vi "KGN Set Pump Mode.vi"(7 "PumpMode-Cluster":T3(array[cluster]) {"concentratio mode" items=["water", "reagent"]; "Reagent" items=["HCl", "HF", "NH3", "HG", "PPM", "ORGANIC"]}, 8 "Fehler (Eingang, kein Fehler)":errorcluster, 9 "Info Cluster":T4, 10 "VISA-Referenz (Eingang)":refnum<visa-resource-name>, 11 "device (Eingang)":u32) -> (0 "Fehler (Ausgang)":errorcluster, 1 "Info Cluster out":T4, 2 "VISA-Referenz (Ausgang)":refnum<visa-resource-name>, 3 "dup device (Ausgang)":u32, 4 "Kommandos gesendet":string[](array[string]))   [LabVIEW 2020, in "Linearisierung v2.lvlib" / "Gasteiler.lvlib" / "HovaCAL_Interface.lvlib" / "KGN.lvlib" / "KGN GUI Set.lvlib"]
uses:
  KGN GUI Set.lvlib
  Controls/Info Cluster.ctl
  Controls/Pump Concentration Mode.ctl
  Controls/Reagent.ctl
  set/set.lvlib
  Controls/Controls.lvlib
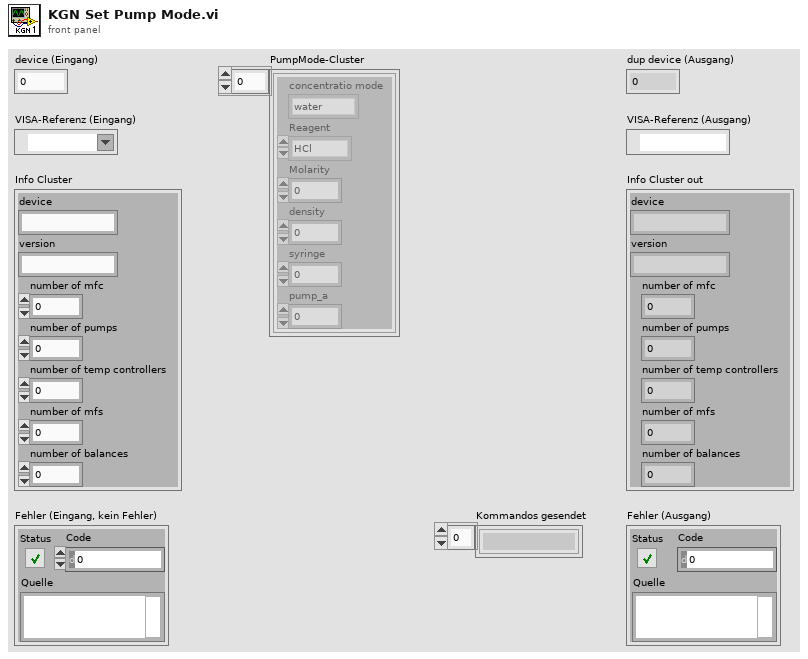
[diagram p1: front panel]
types:
  T1 = typedef "Linearisierung v2.lvlib/Gasteiler.lvlib/HovaCAL_Interface.lvlib/Controls.lvlib/Pump Concentration Mode.ctl" = i32
  T2 = typedef "Linearisierung v2.lvlib/Gasteiler.lvlib/HovaCAL_Interface.lvlib/Controls.lvlib/Reagent.ctl" = i32
  T3 = cluster{"concentratio mode":T1, "Reagent":T2, "Molarity":dbl, "density":dbl, "syringe":dbl, "pump_a":dbl}[]
  T4 = typedef "Linearisierung v2.lvlib/Gasteiler.lvlib/HovaCAL_Interface.lvlib/Controls.lvlib/Info Cluster.ctl" = cluster{"device":string, "version":string, "number of mfc":i32, "number of pumps":i32, "number of temp controllers":i32, "number of mfs":i32, "number of balances":i32}
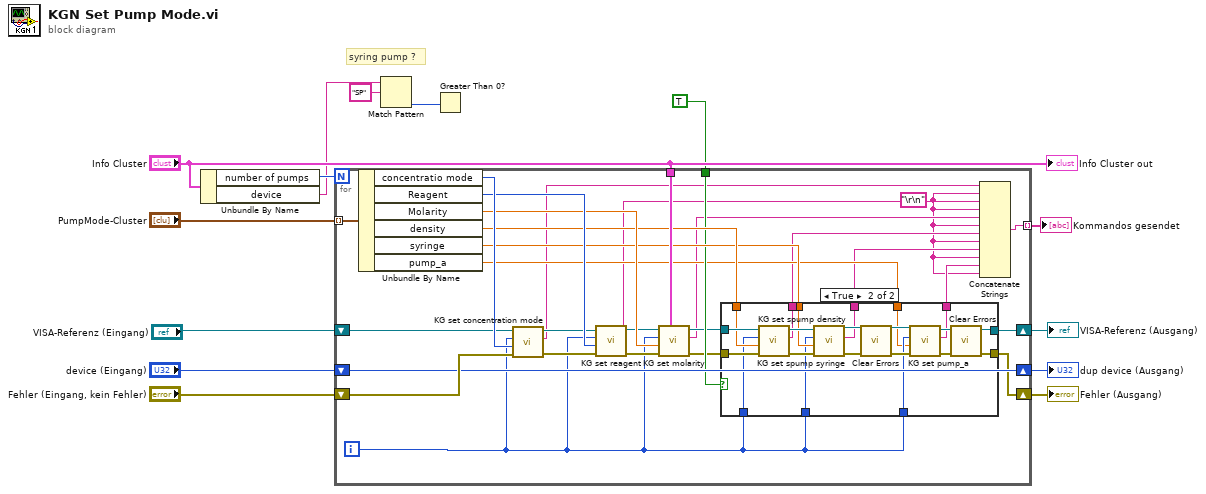
[diagram p0: block diagram]
diagram:
  # "syring pump ?"
  n1 = Unbundle By Name("Info Cluster") -> ("number of pumps"=w9:i32, "device"=w3:string)
  n2 = for {
    N: w9 -> [_]
    tunnel: "PumpMode-Cluster" -> [w42] mode=indexing
    shift-right: [w39] -> w11
    shift-left: "device (Eingang)" -> [w39]
    shift-right: [w38] -> w10
    shift-left: "Fehler (Eingang, kein Fehler)" -> [w43]
    shift-right: [w35] -> w7
    shift-left: "VISA-Referenz (Eingang)" -> [w36]
    tunnel: "Info Cluster" -> [w34]
    tunnel: TRUE -> [w31]
    tunnel: [w16] -> w1 mode=indexing
    i -> [w24]
    w15 = "\r\n"
    n3 = Unbundle By Name(w42) -> ("concentratio mode"=w41:T1, "Reagent"=w40:T2, "Molarity"=w37:dbl, "density"=w33:dbl, "syringe"=w32:dbl, "pump_a"=w23:dbl)
    n4 = call "KG set concentration mode.vi"("Fehler (Eingang, kein Fehler)"=w43, "mode"=w41, "pump"=w24, "VISA-Ressourcenname"=w36) -> ("Fehler (Ausgang)"=w27:errorcluster, "Kommando gesendet"=w22:string, "VISA-Ressourcenname (Ausgang)"=w30:refnum<visa-resource-name>)  [unwired: 5 in]
    n5 = call "KG set reagent.vi"("Fehler (Eingang, kein Fehler)"=w27, "reagent"=w40, "pump"=w24, "VISA-Ressourcenname"=w30) -> ("Fehler (Ausgang)"=w28:errorcluster, "Kommando gesendet"=w21:string, "VISA-Ressourcenname (Ausgang)"=w29:refnum<visa-resource-name>)  [unwired: 5 in]
    n6 = call "KG set molarity.vi"("Info Cluster"=w34, "Fehler (Eingang, kein Fehler)"=w28, "molarity"=w37, "pump"=w24, "VISA-Ressourcenname"=w29) -> ("Fehler (Ausgang)"=w25:errorcluster, "Kommando gesendet"=w20:string, "VISA-Ressourcenname (Ausgang)"=w26:refnum<visa-resource-name>)  [unwired: 4 in]
    n7 = case shown="True" w31 {
      tunnel: [w45 w53] -> w35
      tunnel: w26 -> [w45 w63]
      tunnel: w25 -> [w44 w62]
      tunnel: [w44 w55] -> w38
      tunnel: w33 -> [_ w60]
      tunnel: w32 -> [_ w59]
      tunnel: w24 -> [_ w58]
      tunnel: w24 -> [_ w57]
      tunnel: w24 -> [_ w50]
      tunnel: w23 -> [_ w49]
      tunnel: [_ w48] -> w19
      tunnel: [_ w47] -> w18
      tunnel: [_ w46] -> w17
      frame False {
      }
      frame True {
        n8 = call "KG set spump density.vi"("Fehler (Eingang, kein Fehler)"=w62, "density"=w60, "pump"=w57, "VISA-Ressourcenname"=w63) -> ("Fehler (Ausgang)"=w61:errorcluster, "Kommando gesendet"=w48:string, "VISA-Ressourcenname (Ausgang)"=w64:refnum<visa-resource-name>)  [unwired: 5 in]
        n9 = call "KG set spump syringe.vi"("Fehler (Eingang, kein Fehler)"=w61, "density"=w59, "pump"=w58, "VISA-Ressourcenname"=w64) -> ("Fehler (Ausgang)"=w56:errorcluster, "Kommando gesendet"=w47:string, "VISA-Ressourcenname (Ausgang)"=w54:refnum<visa-resource-name>)  [unwired: 5 in]
        n10 = call <vilib>:"Clear Errors.vi"("error in (no error)"=w56) -> ("error out"=w51:errorcluster)  [unwired: 5 in, 1 out]
        n11 = call "KG set pump_a.vi"("Fehler (Eingang, kein Fehler)"=w51, "A"=w49, "pump"=w50, "VISA-Ressourcenname"=w54) -> ("Fehler (Ausgang)"=w52:errorcluster, "Kommando gesendet"=w46:string, "VISA-Ressourcenname (Ausgang)"=w53:refnum<visa-resource-name>)  [unwired: 5 in]
        n12 = call <vilib>:"Clear Errors.vi"("error in (no error)"=w52) -> ("error out"=w55:errorcluster)  [unwired: 5 in, 1 out]
      }
    }
    n13 = Concatenate Strings(w22, w15, w21, w15, w20, w15, w19, w15, w18, w15, w17, w15) -> (w16:string)
  }
  "dup device (Ausgang)" <- w11
  "Fehler (Ausgang)" <- w10
  "VISA-Referenz (Ausgang)" <- w7
  "Kommandos gesendet" <- w1
  n14 = Match Pattern(string=w3, regular expression="SP" ("Regulärer Ausdruck")) -> (offset past match=w4:i32)  [unwired: 1 in, 3 out]
  n15 = Greater Than 0?(x=w4) -> ()  [unwired: 1 out]
  "Info Cluster out" <- "Info Cluster"
